vi "001 Waveform feed variable.vi"() -> ()   [LabVIEW 2019]
panel:
  in  "stop":bool
  out "Waveform Chart":dbl(graph)
  in  "generació de dades (s)":dbl(knob) scale=0.0..10.0
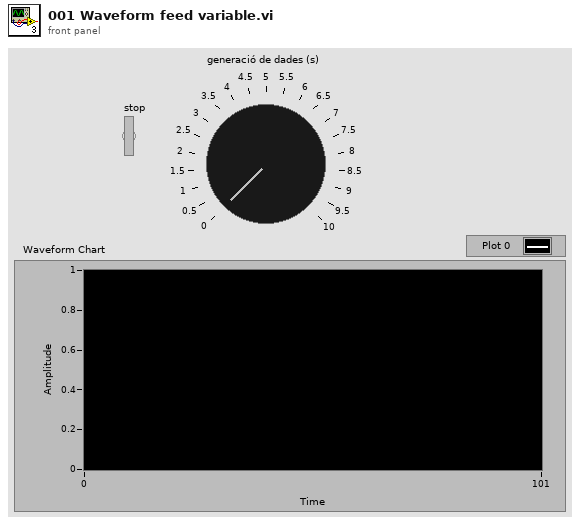
[diagram p1: front panel]
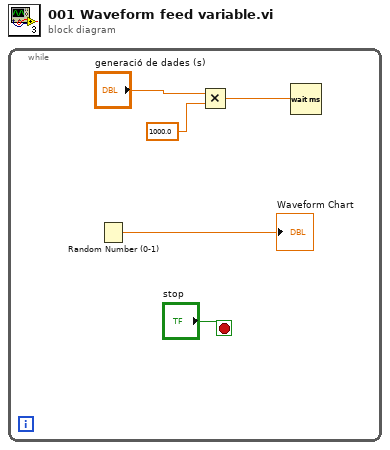
[diagram p0: block diagram]
diagram:
  n1 = while {
    stop <- "stop" stop-if-true
    n2 = Random Number (0-1)() -> (number: 0 to 1=→"Waveform Chart":dbl)
    n3 = Multiply(x="generació de dades (s)", y=1000.0) -> (x*y=w3:dbl)
    n4 = Wait (ms)(milliseconds to wait=w3) -> ()  [unwired: 1 out]
  }
